vi "AllLines.vi"() -> (3 "Lines":i8[][](array[numeric]))   [LabVIEW 2020]
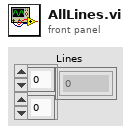
[diagram p1: front panel]
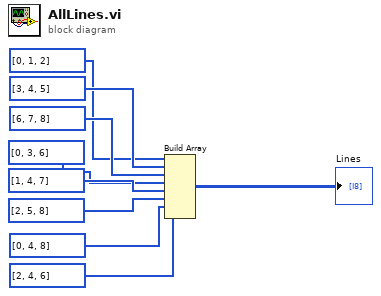
[diagram p0: block diagram]
diagram:
  n1 = Build Array(i8[] [0, 1, 2] ("LineIndices"), i8[] [3, 4, 5] ("LineIndices"), i8[] [6, 7, 8] ("LineIndices"), i8[] [0, 3, 6] ("LineIndices"), i8[] [1, 4, 7] ("LineIndices"), i8[] [2, 5, 8] ("LineIndices"), i8[] [0, 4, 8] ("LineIndices"), i8[] [2, 4, 6] ("LineIndices")) -> (→"Lines":i8[][])
